vi "XY-Data to Dictionary (Multiple).vi"(8 "error in (no error)":errorcluster, 10 "Names":string[](array[string]), 11 "XY-data in":cluster{"X-array":dbl[], "Y-array":dbl[]}[](array[cluster]) {"Y-array" format="%.2p"; "X-array" format="%.2p"}) -> (0 "error out":errorcluster, 3 "Data (Dictionary)":T1[](array[typedef]))   [LabVIEW 2020, in "Data.lvclass"]
uses:
  Data.lvclass
  Typedefs/Dictionary--cluster.ctl
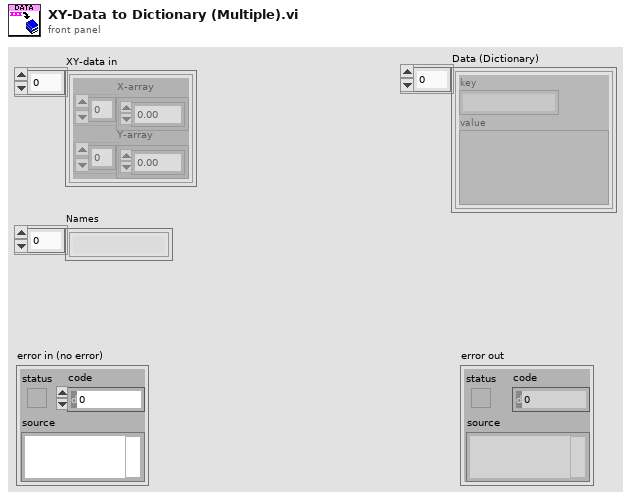
[diagram p1: front panel]
types:
  T1 = typedef "Data.lvclass/Dictionary--cluster.ctl" = cluster{"key":string, "value":variant}
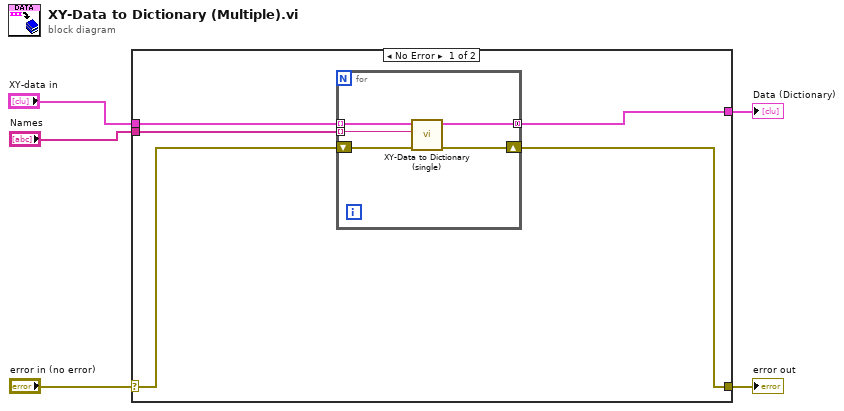
[diagram p0: block diagram]
diagram:
  n1 = case shown="No Error" "error in (no error)" {
    selector: "error in (no error)" -> [w10 w16]
    tunnel: [w9 w16] -> w4
    tunnel: [w6 _] -> w3
    tunnel: "XY-data in" -> [w8 _]
    tunnel: "Names" -> [w7 _]
    frame No Error {
      n2 = for {
        shift-right: [w14] -> w9
        shift-left: w10 -> [w15]
        tunnel: w8 -> [w13] mode=indexing
        tunnel: w7 -> [w12] mode=indexing
        tunnel: [w11] -> w6 mode=concatenating
        n3 = call "XY-Data to Dictionary (single).vi"("error in (no error)"=w15, "Name"=w12, "XY-data in"=w13) -> ("error out"=w14:errorcluster, "Data (Dictionary)"=w11:T1[])  [unwired: 7 in]
      }
    }
    frame Error {
    }
  }
  "error out" <- w4
  "Data (Dictionary)" <- w3
